vi "Digital Input - N Channels - N Samples.vi"() -> ()   [LabVIEW 2019]
uses:
  <vilib>/myRIO/Instrument Drivers/Onboard IO/DI Block/typedefs/DI Block Reference.ctl
  <vilib>/myRIO/Common/Instrument Driver Framework/Utilities/typedefs/myRIO Generic Hardware Reference.ctl
  <vilib>/myRIO/Common/Instrument Driver Framework/Utilities/typedefs/Hardware Version Enum.ctl
  <vilib>/myRIO/Common/Instrument Driver Framework/Utilities/typedefs/myRIO v1.0 Reference.ctl
  <vilib>/myRIO/Common/Instrument Driver Framework/Utilities/typedefs/Generic FPGA Reference.ctl
  <vilib>/myRIO/Common/Instrument Driver Framework/myRIO v1.0/DI Block/typedefs/DI Block Channels List.ctl
  <vilib>/myRIO/Common/Instrument Driver Framework/myRIO v1.0/DI Block/typedefs/DI Block Channels Enum.ctl
  <vilib>/userdefined/High Color/nirio_resource_hc.ctl
  <vilib>/myRIO/Common/Instrument Driver Framework/Utilities/vis/Is FPGA Ref Available.vi
  <vilib>/myRIO/Common/Instrument Driver Framework/ELVIS III v1.0/DI Block/vis/ELVIS III v1.1 Open DI (N Samples).vi
  <vilib>/myRIO/Instrument Drivers/Onboard IO/DI Block/vis/Read.vi
  <vilib>/myRIO/Common/Instrument Driver Framework/Utilities/vis/Validate Channels.vi
  <vilib>/myRIO/Common/Instrument Driver Framework/ELVIS III v1.0/Resource Manager/vis/ELVIS III v1.0 Check For Different Banks.vi
  <vilib>/myRIO/Common/Instrument Driver Framework/ELVIS III v1.0/DI Block/vis/ELVIS III v1.0 DI Block Read.vi
  <vilib>/myRIO/Common/Instrument Driver Framework/myRIO v1.0/UART/vis/myRIO v1.0 Close UART.vi
  <vilib>/myRIO/Common/Instrument Driver Framework/Utilities/vis/Sample Rate To Ticks.vi
  <vilib>/Utility/VariantDataType/GetNumericInfo.vi
  <vilib>/Utility/error.llb/Error Cluster From Error Code.vi
  <vilib>/myRIO/Common/Instrument Driver Framework/ELVIS III v1.0/ELVIS III v1.1 Open.vi
  <vilib>/myRIO/Common/Instrument Driver Framework/ELVIS III v1.0/DI Block/vis/ELVIS III v1.0 Reserve DI Block.vi
  <vilib>/myRIO/Common/Instrument Driver Framework/ELVIS III v1.0/Resource Manager/vis/ELVIS III v1.0 Configure DMAs.vi
  <vilib>/myRIO/Common/Instrument Driver Framework/myRIO v1.0/myRIO v1.0 Close.vi
  <vilib>/myRIO/Common/Instrument Driver Framework/myRIO v1.0/Resource Manager/vis/myRIO v1.0 Block Write Configuration.vi
  <vilib>/myRIO/Common/Instrument Driver Framework/ELVIS III v1.0/DI Block/vis/ELVIS III v1.0 DI Block Read Bank B.vi
  <vilib>/myRIO/Common/Instrument Driver Framework/ELVIS III v1.0/DI Block/vis/ELVIS III v1.0 DI Block Read Bank A.vi
  <vilib>/Waveform/DWDTOps.llb/DWDT Boolean Array to Digital.vi
  <vilib>/myRIO/Common/Instrument Driver Framework/Utilities/vis/FPGA Ref Manager.vi
  <vilib>/myRIO/Common/Instrument Driver Framework/ELVIS III v1.0/ELVIS III v1.0 Reset FPGA.vi
  <vilib>/myRIO/Common/Instrument Driver Framework/myRIO v1.0/IRQ/vis/myRIO v1.0 IRQ Info FGV.vi
  <vilib>/myRIO/Common/Instrument Driver Framework/myRIO v1.0/IRQ/vis/myRIO v1.0 Timer IRQ Info FGV.vi
  <vilib>/myRIO/Common/Instrument Driver Framework/myRIO v1.0/IRQ/vis/myRIO v1.0 ISR Agent.vi
  <vilib>/myRIO/Instrument Drivers/Utilities/vis/Reset Index.vi
  <vilib>/myRIO/Common/Instrument Driver Framework/myRIO v1.0/Resource Manager/vis/myRIO v1.0 Block Write Resource Manager.vi
  <vilib>/myRIO/Express VI/Onboard IO/DI/DI Express VI.xnode
  <vilib>/myRIO/Instrument Drivers/Onboard IO/DI Block/vis/myRIO DI N Samples Open.xnode
  <vilib>/myRIO/Instrument Drivers/Utilities/Utilities.lvlib
  <vilib>/myRIO/Instrument Drivers/Onboard IO/DI Block/DI Block.lvlib
panel:
  in  "Acquire Data":bool
  in  "Stop":bool
  out "Digital Waveform Graph":digitalwaveform(graph)
  # "ELVIS III Control IO"
  # "数字输入N通道"
  # "Overview: Acquires N sample digital data on Bank A, Channels 0 and 1 (A/DIO0 and A/DIO1).\nInstructions:\n1. Connect A/DIO0 and A/DIO1 to valid signals.\n2. Run the VI.\n3. Press Acquire Data to trigger a digital acquisition."
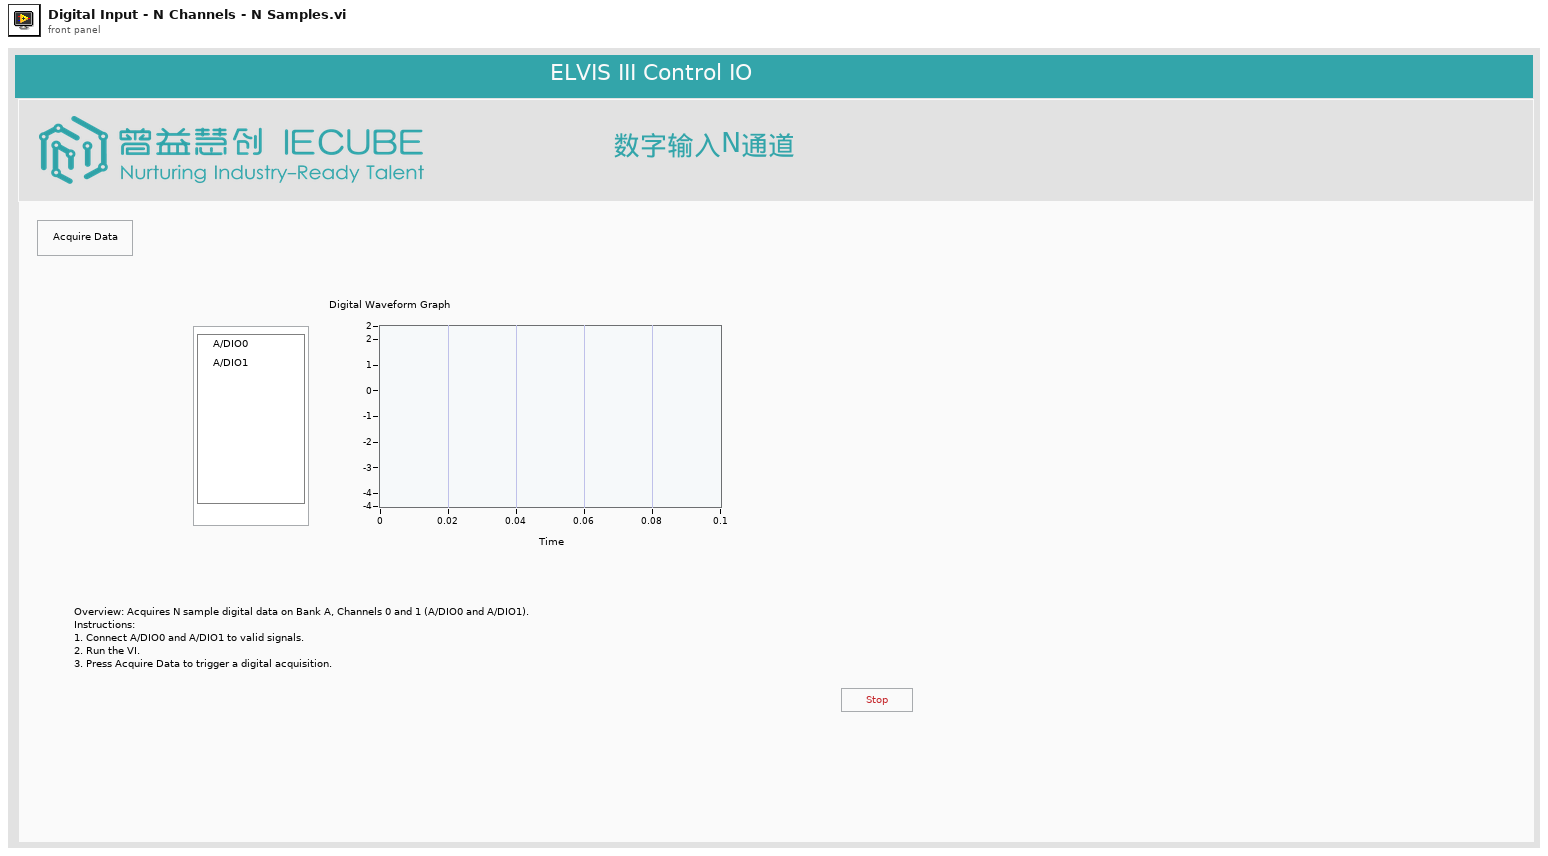
[diagram p1: front panel]
types:
  T1 = typedef "DI Block.lvlib/DI Block Reference.ctl" = cluster{"myRIO Reference":T2, "DI (N Samples) Channels List":T6}
  T2 = typedef "myRIO Generic Hardware Reference.ctl" = cluster{"myRIO Model":T3, "myRIO Hardware Reference":T4}
  T3 = typedef "Hardware Version Enum.ctl" = enum16{"Unknown", "myRIO-1900", "myRIO-1950", "roboRIO", "NI ELVIS RIO CM", "ELVIS III"}
  T4 = typedef "myRIO v1.0 Reference.ctl" = cluster{"Generic FPGA Reference":T5, "Allow multiple opens":bool}
  T5 = typedef "Generic FPGA Reference.ctl" = refnum<k20>
  T6 = typedef "DI Block Channels List.ctl" = T7[]
  T7 = typedef "DI Block Channels Enum.ctl" = enum16{"Not Connected", "A/DI0 (N Samples)", "A/DI1 (N Samples)", "A/DI2 (N Samples)", "A/DI3 (N Samples)", "A/DI4 (N Samples)", "A/DI5 (N Samples)", "A/DI6 (N Samples)", "A/DI7 (N Samples)", "A/DI8 (N Samples)", "A/DI9 (N Samples)", "A/DI10 (N Samples)", "A/DI11 (N Samples)", "A/DI12 (N Samples)", "A/DI13 (N Samples)", "A/DI14 (N Samples)", "A/DI15 (N Samples)", "A/DI16 (N Samples)", "A/DI17 (N Samples)", "A/DI18 (N Samples)", "A/DI19 (N Samples)", "B/DI0 (N Samples)", "B/DI1 (N Samples)", "B/DI2 (N Samples)", "B/DI3 (N Samples)", "B/DI4 (N Samples)", "B/DI5 (N Samples)", "B/DI6 (N Samples)", "B/DI7 (N Samples)", "B/DI8 (N Samples)", "B/DI9 (N Samples)", "B/DI10 (N Samples)", "B/DI11 (N Samples)", "B/DI12 (N Samples)", "B/DI13 (N Samples)", "B/DI14 (N Samples)", "B/DI15 (N Samples)", "B/DI16 (N Samples)", "B/DI17 (N Samples)", "B/DI18 (N Samples)", "B/DI19 (N Samples)"}
  T8 = typedef "nirio_resource_hc.ctl" = tag
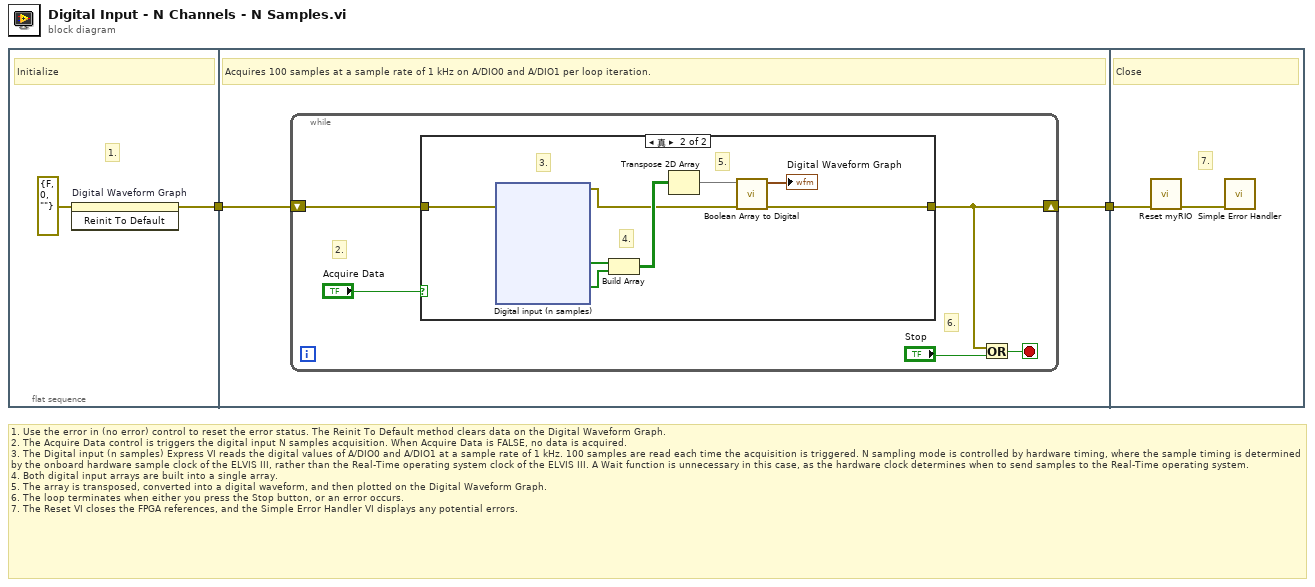
[diagram p0: block diagram]
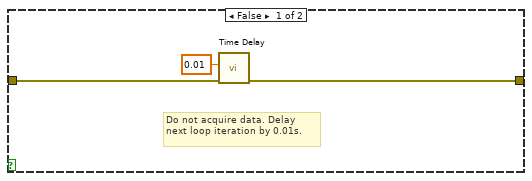
[diagram p2: hidden frame]
diagram:
  # "1. Use the error in (no error) control to reset the error status. The Reinit To Default method clears data on the Digital Waveform Graph.\n2. The Acquire Data control is triggers the digital input N samples acquisition. When Acquire Data is FALSE, no data is acquired.\n3. The Digital input (n samples) Express VI reads the digital values of A/DIO0 and A/DIO1 at a sample rate of 1 kHz. 100 samples are read each time the acquisition is triggered. N sampling mode is controlled by hardware timing, where the sample timing is determined by the onboard hardware sample clock of the ELVIS III, rather than the Real-Time operating system clock of the ELVIS III. A Wait function is unnecessary in this case, as the hardware clock determines when to send samples to the Real-Time operating system.\n4. Both digital input arrays are built into a single array.\n5. The array is transposed, converted into a digital waveform, and then plotted on the Digital Waveform Graph.\n6. The loop terminates when either you press the Stop button, or an error occurs.\n7. The Reset VI closes the FPGA references, and the Simple Error Handler VI displays any potential errors."
  n1 = flat-sequence {
    tunnel: [w3] -> w1
    tunnel: [w6] -> w2
    tunnel: w1 -> [w5]
    tunnel: w2 -> [w62]
    frame #0 {
      # "1."
      # "Initialize"
      n2 = invoke on="Digital Waveform Graph" class="DigitalGraph (strict)" method="Reinit To Default"(error in=errorcluster {"status"=FALSE, "code"=0, "source"=""} ("Error In")) -> (error out=w3:errorcluster)  [unwired: 2 in, 2 out]
    }
    frame #1 {
      # "Acquires 100 samples at a sample rate of 1 kHz on A/DIO0 and A/DIO1 per loop iteration."
      n3 = while {
        shift-right: [w9] -> w6
        shift-left: w5 -> [w10]
        stop <- w11 stop-if-true
        # "6."
        # "2."
        n4 = case shown="真" "Acquire Data" {
          tunnel: w10 -> [w13 w22]
          tunnel: [w12 w18] -> w9
          frame False {
            # "Do not acquire data. Delay next loop iteration by 0.01s."
            n5 = call "Time Delay"("error in (no error)"=w13, "Delay Time (s)"=0.01) -> ("error out"=w12:errorcluster)  [unwired: 9 in]
          }
          frame True {
            # "5."
            # "4."
            # "3."
            n6 = xnode "Digital input (n samples)"("error in (no error)"=w22) -> ("A/DI0 (N Samples)"=w21:bool[], "A/DI1 (N Samples)"=w20:bool[], "error out"=w17:errorcluster)
            n7 = Build Array(w21, w20) -> (w19:bool[][])
            n8 = Transpose 2D Array(2D array=w19) -> (transposed array=w15:bool[][])
            n9 = call-poly <vilib>:"Boolean Array to Digital.vi"("error in (no error)"=w17, "boolean array"=w15) -> ("error out"=w18:errorcluster, "digital waveform"=→"Digital Waveform Graph":digitalwaveform)  [unwired: 8 in]
          }
        }
        n10 = Or(x=w9, y="Stop") -> (x .or. y?=w11:bool)
      }
    }
    frame #2 {
      # "7."
      # "Close"
      n11 = call <vilib>:"Reset myRIO.vi"("error in (no error)"=w62) -> ("error out"=w61:errorcluster)  [unwired: 10 in]
      n12 = call <vilib>:"Simple Error Handler.vi"("error in (no error)"=w61) -> ()  [unwired: 4 in, 5 out]
    }
  }
